vi "DAE Radau 5th Order.vi"   [LabVIEW 2020, in "NI_DAE.lvlib"]
doc: "Solves differential algebraic equations (DAEs) with initial conditions by using the Radau IIA method. You must manually select the polymorphic instance to use."
uses:
  <vilib>/gmath/NI_DAE.lvlib
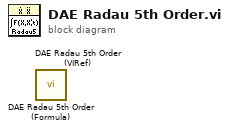
[diagram p0: block diagram]
diagram:
  n1 = call <vilib>:"DAE Radau 5th Order (Formula).vi"() -> ()  [unwired: 8 in, 4 out]
  n2 = call <vilib>:"DAE Radau 5th Order (VIRef).vi"() -> ()  [unwired: 8 in, 4 out]
